vi "RANGE Flow Rate Calculation.vi"(8 "Error In":errorcluster, 9 "Heating Value (BTU/ft³)":dbl, 10 "Flow Rate Factor":dbl, 11 "Ft³/HR":dbl) -> (0 "Error Out":errorcluster, 3 "Flow Rate (BTU/Hr)":dbl)   [LabVIEW 2018]
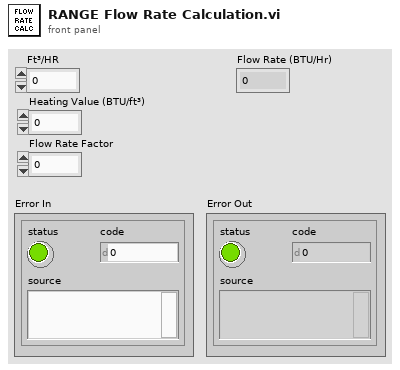
[diagram p1: front panel]
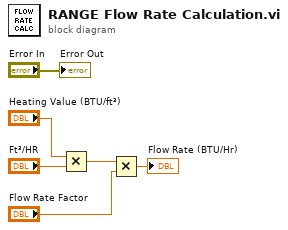
[diagram p0: block diagram]
diagram:
  n1 = Multiply(x="Heating Value (BTU/ft³)", y="Ft³/HR") -> (x*y=w3:dbl)
  n2 = Multiply(x=w3, y="Flow Rate Factor") -> (x*y=→"Flow Rate (BTU/Hr)":dbl)
  "Error Out" <- "Error In"
